vi "setup_for_move.vi"(7 "USB setting for move":cluster{"S/N":string, "USB Search?":bool}={"S/N"="0135500392", "USB Search?"=FALSE}, 8 "错误输入（无错误）":errorcluster, 9 "System no.输入":i32=1 min=1 step=1, 10 "DaisyChain setting for move":T2={"Register DC"=FALSE, "DaisyChain Search?"=TRUE, "Device ID"=1}, 11 "RON settings":T1={"RON Affected axes"=[], "Reference mode"=[], "Check FRF?"=TRUE}) -> (0 "错误输出":errorcluster, 2 "Conn. \nAxes":string[](array[string]), 3 "System no.输出":i32)   [LabVIEW 2017]
panel:
  out "Device ID out":i32
  in  "Axes to move":string[](array[string])
  out "SN out":string
  out "Identification":string
  out "Position":dbl[](array[numeric]) format="%.6f"
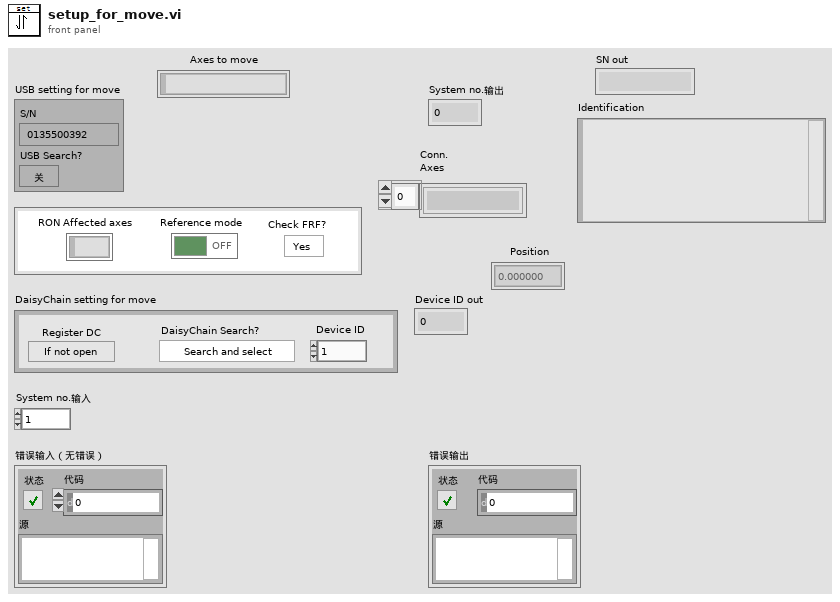
[diagram p1: front panel]
types:
  T1 = cluster{"RON Affected axes":string[], "Reference mode":bool[], "Check FRF?":bool}
  T2 = cluster{"Register DC":bool, "DaisyChain Search?":bool, "Device ID":i32}
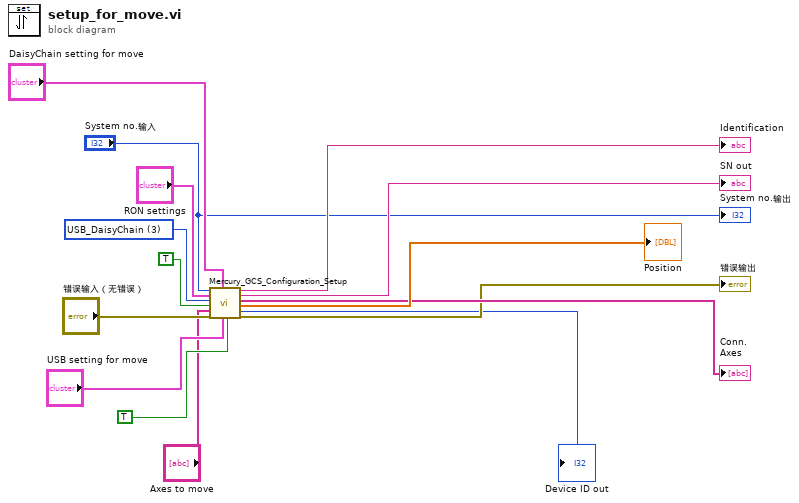
[diagram p0: block diagram]
diagram:
  w9 = u16 3 items=["RS232", "RS232 DaisyChain", "USB", "USB_DaisyChain"] ("Interface")
  n1 = call "Mercury_GCS_Configuration_Setup.vi"("System no."="System no.输入", "RON settings"="RON settings", "Interface"=w9, "All axes?"=TRUE ("Switch servo on?"), "Axes to move"="Axes to move", "error in"="错误输入（无错误）", "DaisyChain settings"="DaisyChain setting for move", "USB settings"="USB setting for move", "Switch servo on?"=TRUE) -> ("Device ID out"=→"Device ID out":i32, "Identification"=→"Identification":string, "SN out"=→"SN out":string, "Conn. \nAxes"=→"Conn. \nAxes":string[], "Position"=→"Position":dbl[], "error out"=→"错误输出":errorcluster)  [unwired: 4 in, 1 out]
  "System no.输出" <- "System no.输入"
